vi "Read Stream Specification.vi"(8 "error in (no error)":errorcluster, 11 "Stream in":refnum<class "Stream.lvclass">) -> (0 "error out":errorcluster, 2 "Stream Specification":T1, 3 "Stream":refnum<class "Stream.lvclass">)   [LabVIEW 2020, in "capture.lvlib" / "Stream.lvclass"]
doc: "Read Stream Specification."
uses:
  Stream.lvclass
  Stream Specification.ctl
  common/Image Size (Integer).ctl
  Frames per Second.ctl
  Stream.lvclass/Stream.ctl
  common/common.lvlib
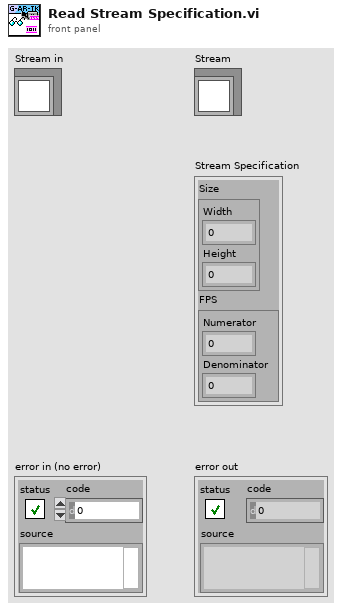
[diagram p1: front panel]
types:
  T1 = typedef "capture.lvlib/Stream.lvclass/Stream Specification.ctl" = cluster{"Size":T2, "FPS":T3}
  T2 = typedef "common.lvlib/Image Size (Integer).ctl" = cluster{"Width":u16, "Height":u16}
  T3 = typedef "capture.lvlib/Stream.lvclass/Frames per Second.ctl" = cluster{"Numerator":u32, "Denominator":u32}
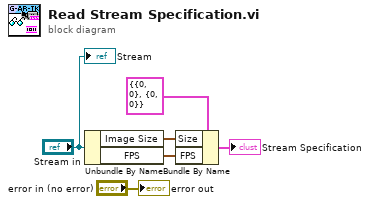
[diagram p0: block diagram]
diagram:
  n1 = Unbundle By Name("Stream in") -> ("Image Size"=w2:T2, "FPS"=w1:T3)
  n2 = Bundle By Name(cluster=T1 {"Size"={"Width"=0, "Height"=0}, "FPS"={"Numerator"=0, "Denominator"=0}} ("Desired Stream Specification"), "Size"=w2, "FPS"=w1) -> (→"Stream Specification":T1)
  "error out" <- "error in (no error)"
  "Stream" <- "Stream in"
